vi "Get Sender.vi"(11 "Message":refnum<class "Message.lvclass">) -> (2 "Sender":string, 3 "Message":refnum<class "Message.lvclass">)   [LabVIEW 2017, in "LapDog.Messaging.v3.lvlib" / "Message.lvclass"]
uses:
  Message.lvclass
  Message.lvclass/Message.ctl
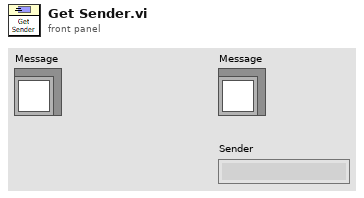
[diagram p1: front panel]
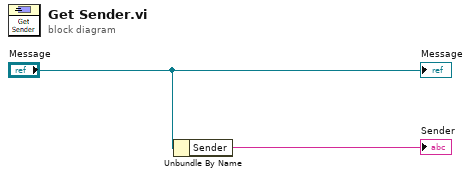
[diagram p0: block diagram]
diagram:
  n1 = Unbundle By Name("Message") -> ("Sender"=→"Sender":string)
  "Message" <- "Message"
